vi "Change Database.vi"(8 "error in (no error)":errorcluster, 11 "Node Ptr":u64 format="%.0x") -> (0 "error out":errorcluster)   [LabVIEW 2025, in "Protection and Counter Addon System Explorer.lvlib"]
uses:
  Protection and Counter Addon System Explorer.lvlib
  Types/Base Frame Info.ctl
  <vilib>/NI VeriStand/Custom Device API/Custom Device Item Ref.ctl
  Types/CAN Filter Type.ctl
  <vilib>/NI VeriStand/Custom Device Tools/Custom Device Utility Library/Search Direction.ctl
  <vilib>/NI VeriStand/Custom Device API/Custom Device Channel.ctl
  <vilib>/NI VeriStand/Custom Device API/Custom Device Channel Type.ctl
  Addon Shared/SubVIs/GUID Lookup.vi
  <vilib>/NI/NI VeriStand Advanced SysDef API/_SubVIs/SysDef.Search.GUIDs.vi
  <vilib>/NI VeriStand/Custom Device API/Get Item Property (U32).vi
  <vilib>/NI VeriStand/Custom Device Tools/Custom Device Utility Library/NI VeriStand - Search for Item by GUID.vi
  <vilib>/NI/NI VeriStand Advanced SysDef API/_SubVIs/SysDef.Property.Set.U32.vi
  <vilib>/NI/NI VeriStand Advanced SysDef API/_SubVIs/SysDef.Search.Name.vi
  Addon Shared/Protection and Counter Addon Shared.lvlib
  <vilib>/NI/NI VeriStand Advanced SysDef API/SysDef API/Advanced System Definition.lvlib
  <vilib>/NI VeriStand/Custom Device API/Custom Device API.lvlib
  <resource>/objmgr/xnet.rc
  <vilib>/NI VeriStand/Custom Device Tools/Custom Device Utility Library/Custom Device Utility Library.lvlib
panel:
  in  "Tag":string
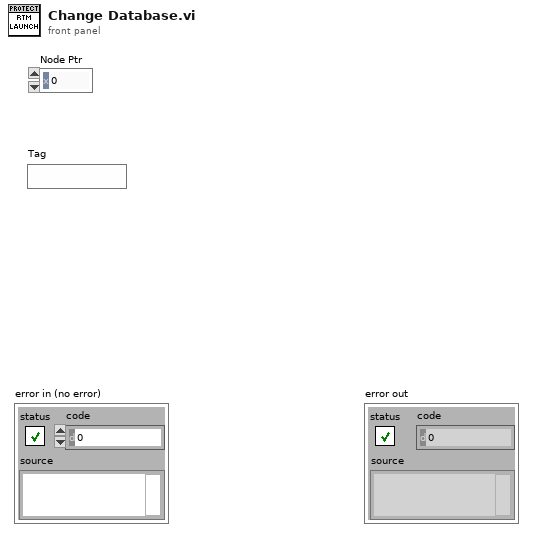
[diagram p1: front panel]
types:
  T1 = typedef "Protection and Counter Addon System Explorer.lvlib/Base Frame Info.ctl" = cluster{"Name":string, "ID":u32, "Signals":string[], "Node Ref":T2, "Type":T3}
  T2 = typedef "Custom Device API.lvlib/Custom Device Item Ref.ctl" = u64
  T3 = typedef "Protection and Counter Addon System Explorer.lvlib/CAN Filter Type.ctl" = enum16{"Cyclic Data", "Event Data", "Cyclic/Event", "All"}
  T4 = typedef "Custom Device API.lvlib/Custom Device Item Info.ctl" = cluster{"Name":string, "Is Channel":bool, "GUID":string, "Is Waveform":bool}
  T5 = typedef "Protection and Counter Addon Shared.lvlib/XNET Settings.ctl" = cluster{"Database":refnum<k21>, "Cluster":refnum<k21>, "Port":string, "Baud rate [Bd]":u64, "Termination":u32, "CAN I/O Mode":u32, "FD Baud rate [Bd]":u64, "Priority":i32, "Use Legacy":bool, "FD ISO Mode":u32, "Default Max Counter Value":dbl, "Default Protect Type":T6}
  T6 = typedef "Protection and Counter Support Shared.lvlib/Protection Type.ctl" = enum16{"Arb ID + Bytes Checksum with Inversion", "Arb ID + Bytes CRC with Inversion", "Reversed Raw Signal Checksum with Inversion", "Concatenated Two's Compliment"}
  T7 = typedef "Protection and Counter Addon System Explorer.lvlib/CAN Update Results.ctl" = cluster{"Frames to Delete":T2[], "Frames to Update":T8[], "New Cluster":refnum<k21>, "Frames to Add":T9[]}
  T8 = typedef "Protection and Counter Addon System Explorer.lvlib/CAN Frame Update Results.ctl" = cluster{"Node Ref":T2, "Name":string, "ID":u32, "New Signals":string[], "Delete Signals":string[], "Type":T3}
  T9 = typedef "Protection and Counter Addon System Explorer.lvlib/Base Frame Info_NoVS.ctl" = cluster{"Name":string, "ID":u32, "Signals":string[], "Type":T3}
  T10 = typedef "Custom Device Utility Library.lvlib/Search Direction.ctl" = enum16{"Down", "Up"}
  T11 = typedef "Custom Device API.lvlib/Custom Device Channel.ctl" = cluster{"Type":T12, "Units":string, "Default Value":dbl, "Faultable":bool, "Scalable":bool}
  T12 = typedef "Custom Device API.lvlib/Custom Device Channel Type.ctl" = enum16{"Input", "Output"}
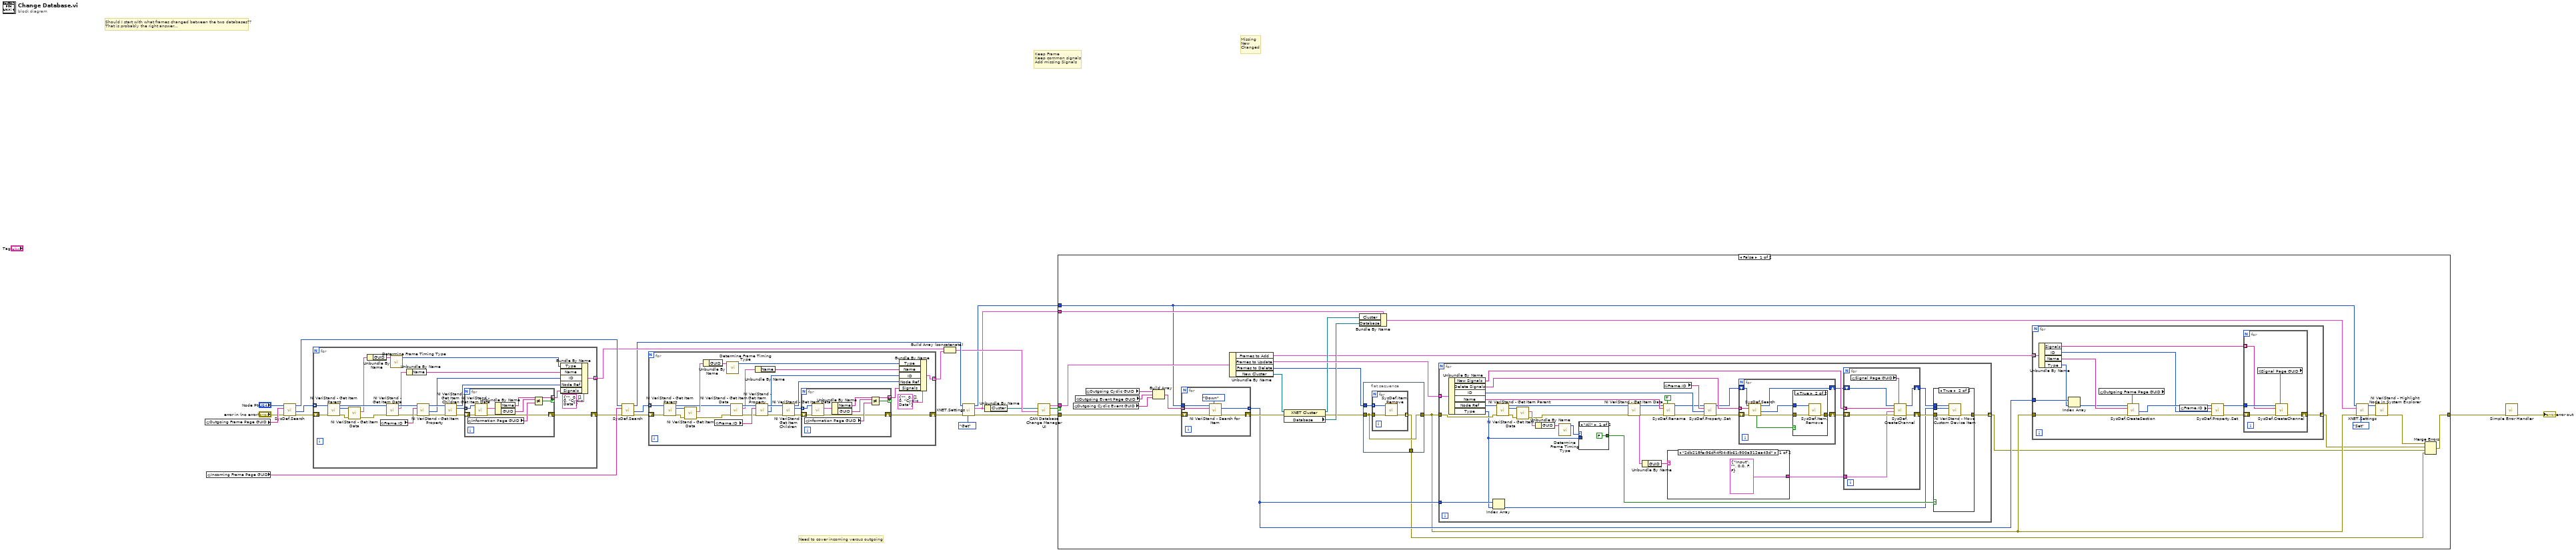
[diagram p0: block diagram]
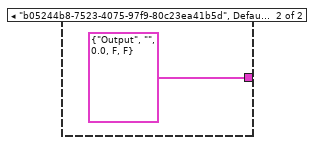
[diagram p4: hidden frame]
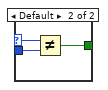
[diagram p5: hidden frame]
diagram:
  # "Missing\nNew\nChanged"
  # "Should I start with what frames changed between the two databases??\nThat is probably the right answer..."
  # "Keep Frame\nKeep common signals\nAdd missing Signals"
  # "Need to cover incoming versus outgoing"
  n1 = global read "GUID Lookup.vi" "Outgoing Frame Page GUID"() -> (w25:string)
  n2 = global read "GUID Lookup.vi" "Incoming Frame Page GUID"() -> (w24:string)
  n3 = call-poly <vilib>:"SysDef.Search.vi"("error in (no error)"="error in (no error)", "GUID"=w25, "nodeID"="Node Ptr") -> ("error out"=w23:errorcluster, "Values Out"=w22:u64[], "nodeID out"=w18:u64)  [unwired: 5 in, 1 out]
  n4 = for {
    tunnel: w22 -> [w33] mode=indexing
    tunnel: [w39] -> w17 mode=indexing
    shift-right: [w38] -> w19
    shift-left: w23 -> [w32]
    n5 = call <vilib>:"NI VeriStand - Get Item Parent.vi"("error in (no error)"=w32, "Item Ref in"=w33) -> ("error out"=w30:errorcluster, "Parent Ref"=w31:T2, "Item Ref out"=w34:T2)  [unwired: 6 in, 1 out]
    n6 = call <vilib>:"NI VeriStand - Get Item Data.vi"("error in (no error)"=w30, "Item Ref in"=w31) -> ("error out"=w29:errorcluster, "Item Info"=w28:T4)  [unwired: 6 in, 2 out]
    n7 = Unbundle By Name(w28) -> ("GUID"=w27:string)
    n8 = global read "GUID Lookup.vi" "Frame.ID"() -> (w47:string)
    n9 = call <vilib>:"NI VeriStand - Get Item Data.vi"("error in (no error)"=w29, "Item Ref in"=w34) -> ("error out"=w44:errorcluster, "Item Info"=w42:T4, "Item Ref out"=w43:T2)  [unwired: 6 in, 1 out]
    n10 = call "Determine Frame Timing Type.vi"("GUID"=w27) -> ("CAN:Frame Type"=w26:T3)  [unwired: 10 in]
    n11 = Unbundle By Name(w42) -> ("Name"=w36:string)
    n12 = call-poly <vilib>:"NI VeriStand - Get Item Property.vi"("error in (no error)"=w44, "Property Name"=w47, "Item Ref in"=w43) -> ("error out"=w48:errorcluster, "Value"=w41:u32, "Item Ref out"=w49:T2)  [unwired: 5 in, 1 out]
    n13 = call <vilib>:"NI VeriStand - Get Item Children.vi"("error in (no error)"=w48, "Item Ref in"=w49) -> ("error out"=w45:errorcluster, "Child Refs"=w46:T2[], "Item Ref out"=w35:T2)  [unwired: 6 in, 1 out]
    n14 = for {
      tunnel: w46 -> [w57] mode=indexing
      shift-right: [w52] -> w38
      shift-left: w45 -> [w56]
      tunnel: [w50] -> w40 mode=indexing if=w51
      n15 = global read "GUID Lookup.vi" "Information Page GUID"() -> (w54:string)
      n16 = call <vilib>:"NI VeriStand - Get Item Data.vi"("error in (no error)"=w56, "Item Ref in"=w57) -> ("error out"=w52:errorcluster, "Item Info"=w55:T4)  [unwired: 6 in, 2 out]
      n17 = Unbundle By Name(w55) -> ("Name"=w50:string, "GUID"=w53:string)
      n18 = Not Equal?(x=w53, y=w54) -> (x != y?=w51:bool)
    }
    n19 = Bundle By Name(cluster=T1 {"Name"="", "ID"=0, "Signals"=[], "Node Ref"=0, "Type"=enum."Cyclic Data"}, "Type"=w26, "Name"=w36, "ID"=w41, "Node Ref"=w35, "Signals"=w40) -> (w39:T1)
  }
  n20 = call-poly <vilib>:"SysDef.Search.vi"("error in (no error)"=w19, "GUID"=w24, "nodeID"=w18) -> ("error out"=w20:errorcluster, "Values Out"=w21:u64[], "nodeID out"=w8:u64)  [unwired: 5 in, 1 out]
  n21 = for {
    tunnel: w21 -> [w61] mode=indexing
    shift-right: [w70] -> w9
    shift-left: w20 -> [w62]
    tunnel: [w69] -> w16 mode=indexing
    n22 = call <vilib>:"NI VeriStand - Get Item Parent.vi"("error in (no error)"=w62, "Item Ref in"=w61) -> ("error out"=w65:errorcluster, "Parent Ref"=w66:T2, "Item Ref out"=w59:T2)  [unwired: 6 in, 1 out]
    n23 = call <vilib>:"NI VeriStand - Get Item Data.vi"("error in (no error)"=w65, "Item Ref in"=w66) -> ("error out"=w60:errorcluster, "Item Info"=w64:T4)  [unwired: 6 in, 2 out]
    n24 = Unbundle By Name(w64) -> ("GUID"=w63:string)
    n25 = global read "GUID Lookup.vi" "Frame.ID"() -> (w79:string)
    n26 = call "Determine Frame Timing Type.vi"("GUID"=w63) -> ("CAN:Frame Type"=w58:T3)  [unwired: 10 in]
    n27 = call <vilib>:"NI VeriStand - Get Item Data.vi"("error in (no error)"=w60, "Item Ref in"=w59) -> ("error out"=w78:errorcluster, "Item Info"=w72:T4, "Item Ref out"=w76:T2)  [unwired: 6 in, 1 out]
    n28 = Unbundle By Name(w72) -> ("Name"=w71:string)
    n29 = call-poly <vilib>:"NI VeriStand - Get Item Property.vi"("error in (no error)"=w78, "Property Name"=w79, "Item Ref in"=w76) -> ("error out"=w77:errorcluster, "Value"=w73:u32, "Item Ref out"=w75:T2)  [unwired: 5 in, 1 out]
    n30 = call <vilib>:"NI VeriStand - Get Item Children.vi"("error in (no error)"=w77, "Item Ref in"=w75) -> ("error out"=w80:errorcluster, "Child Refs"=w81:T2[], "Item Ref out"=w67:T2)  [unwired: 6 in, 1 out]
    n31 = for {
      tunnel: w81 -> [w89] mode=indexing
      shift-right: [w84] -> w70
      shift-left: w80 -> [w88]
      tunnel: [w82] -> w74 mode=indexing if=w83
      n32 = global read "GUID Lookup.vi" "Information Page GUID"() -> (w86:string)
      n33 = call <vilib>:"NI VeriStand - Get Item Data.vi"("error in (no error)"=w88, "Item Ref in"=w89) -> ("error out"=w84:errorcluster, "Item Info"=w87:T4)  [unwired: 6 in, 2 out]
      n34 = Unbundle By Name(w87) -> ("Name"=w82:string, "GUID"=w85:string)
      n35 = Not Equal?(x=w85, y=w86) -> (x != y?=w83:bool)
    }
    n36 = Bundle By Name(cluster=T1 {"Name"="", "ID"=0, "Signals"=[], "Node Ref"=0, "Type"=enum."Cyclic Data"}, "Type"=w58, "Name"=w71, "ID"=w73, "Node Ref"=w67, "Signals"=w74) -> (w69:T1)
  }
  n37 = Build Array (concatenate)(w17, w16) -> (w6:T1[])
  n38 = call "XNET.Settings.vi"("Action"=enum8{"Get", "Set"}."Get", "error in (no error)"=w9, "Parent Ref in"=w8) -> ("error out"=w5:errorcluster, "XNET Settings"=w3:T5, "Item Ref out"=w2:T2)  [unwired: 6 in]
  n39 = Unbundle By Name(w3) -> ("Cluster"=w4:refnum<k21>)
  n40 = call "CAN Database Change Manager UI.vi"("error in (no error)"=w5, "VS Existing Frames"=w6, "Old Cluster"=w4) -> ("error out"=w13:errorcluster, "Cancel Out"=w12:bool, "CAN Update"=w11:T7)  [unwired: 6 in]
  n41 = case shown="False" w12 {
    tunnel: w13 -> [w101 w213]
    tunnel: w11 -> [w116 _]
    tunnel: [w90 w213] -> w10
    tunnel: w3 -> [w113 _]
    tunnel: w2 -> [w104 _]
    frame False {
      n42 = global read "GUID Lookup.vi" "Outgoing Cyclic Event GUID"() -> (w105:string)
      n43 = global read "GUID Lookup.vi" "Outgoing Event Page GUID"() -> (w106:string)
      n44 = global read "GUID Lookup.vi" "Outgoing Cyclic GUID"() -> (w107:string)
      n45 = Build Array(w107, w106, w105) -> (w103:string[])
      n46 = for {
        tunnel: w104 -> [w127]
        tunnel: w103 -> [w126] mode=indexing
        shift-right: [w124] -> w102
        shift-left: w101 -> [w125]
        tunnel: [w123] -> w97 mode=indexing
        n47 = call-poly <vilib>:"NI VeriStand - Search for Item.vi"("Direction (Down)"=Search_Direction."Down", "error in"=w125, "Item GUID"=w126, "Section Ref in"=w127) -> ("error out"=w124:errorcluster, "Item Ref"=w123:T2)  [unwired: 4 in, 2 out]
      }
      n48 = Unbundle By Name(w116) -> ("Frames to Add"=w98:T9[], "Frames to Update"=w115:T8[], "Frames to Delete"=w99:T2[], "New Cluster"=w100:refnum<k21>)
      n49 = property class="XNET Cluster"(reference=w100, error in=w102) -> (reference out=w112:refnum<k21>, error out=w96:errorcluster, "Database"=w111:refnum<k21>)
      n50 = Bundle By Name(cluster=w113, "Cluster"=w112, "Database"=w111) -> (w110:T5)
      n51 = flat-sequence {
        tunnel: w99 -> [w119]
        tunnel: w96 -> [w118]
        tunnel: [w118] -> w95
        tunnel: [w117] -> w92
        frame #0 {
          n52 = for {
            tunnel: w119 -> [w120] mode=indexing
            tunnel: w118 -> [w122]
            tunnel: [w121] -> w117 mode=indexing
            n53 = call <vilib>:"SysDef.Item.Remove.vi"("error in (no error)"=w122, "nodeID"=w120) -> ("error out"=w121:errorcluster)  [unwired: 8 in, 1 out]
          }
        }
      }
      n54 = for {
        tunnel: w115 -> [w162] mode=indexing
        tunnel: w97 -> [w147]
        tunnel: w95 -> [w150]
        tunnel: [w132] -> w93 mode=indexing
        n55 = Unbundle By Name(w162) -> ("New Signals"=w157:string[], "Delete Signals"=w158:string[], "ID"=w160:u32, "Name"=w161:string, "Node Ref"=w152:T2, "Type"=w146:T3)
        n56 = Index Array(array=w147, index=w146) -> (element=w130:T2)
        n57 = call <vilib>:"NI VeriStand - Get Item Parent.vi"("error in (no error)"=w150, "Item Ref in"=w152) -> ("error out"=w155:errorcluster, "Parent Ref"=w156:T2, "Item Ref out"=w151:T2)  [unwired: 6 in, 1 out]
        n58 = call <vilib>:"NI VeriStand - Get Item Data.vi"("error in (no error)"=w155, "Item Ref in"=w156) -> ("error out"=w149:errorcluster, "Item Info"=w154:T4)  [unwired: 6 in, 2 out]
        n59 = Unbundle By Name(w154) -> ("GUID"=w153:string)
        n60 = call "Determine Frame Timing Type.vi"("GUID"=w153) -> ("CAN:Frame Type"=w148:T3)  [unwired: 10 in]
        n61 = case shown="\"All\"" w148 {
          selector: w148 -> [_ w190]
          tunnel: w146 -> [_ w192]
          tunnel: [FALSE w191] -> w131
          frame "All" {
          }
          frame Default {
            n62 = Not Equal?(x=w190, y=w192) -> (x != y?=w191:bool)
          }
        }
        n63 = call <vilib>:"NI VeriStand - Get Item Data.vi"("error in (no error)"=w149, "Item Ref in"=w151) -> ("error out"=w139:errorcluster, "Item Info"=w138:T4, "Item Ref out"=w140:T2)  [unwired: 6 in, 1 out]
        n64 = Unbundle By Name(w138) -> ("GUID"=w137:string)
        n65 = call <vilib>:"SysDef.Rename.vi"("Force Rename (F)"=TRUE, "error in (no error)"=w139, "Name"=w161, "nodeID"=w140) -> ("error out"=w144:errorcluster, "nodeID out"=w145:u64)  [unwired: 5 in, 1 out]
        n66 = global read "GUID Lookup.vi" "Frame.ID"() -> (w159:string)
        n67 = case shown="\"2db218fe-96df-4f04-8b61-900a312ea43d\"" w137 {
          tunnel: [T11 {"Type"=enum."Input", "Units"="", "Default Value"=0.0, "Faultable"=FALSE, "Scalable"=FALSE} ("Channel") T11 {"Type"=enum."Output", "Units"="", "Default Value"=0.0, "Faultable"=FALSE, "Scalable"=FALSE} ("Channel")] -> w136
          frame "2db218fe-96df-4f04-8b61-900a312ea43d" {
          }
          frame "b05244b8-7523-4075-97f9-80c23ea41b5d", Default {
          }
        }
        n68 = call-poly <vilib>:"SysDef.Property.Set.vi"("error in (no error)"=w144, "Value"=w160, "Property Name"=w159, "nodeID"=w145) -> ("error out"=w135:errorcluster, "nodeID out"=w143:u64)  [unwired: 6 in]
        n69 = for {
          tunnel: w158 -> [w175] mode=indexing
          shift-right: [w178] -> w142
          shift-left: w143 -> [w182]
          shift-right: [w177] -> w141
          shift-left: w135 -> [w176]
          n70 = call-poly <vilib>:"SysDef.Search.vi"("error in (no error)"=w176, "Name"=w175, "nodeID"=w182) -> ("error out"=w179:errorcluster, "Value out"=w180:u64, "nodeID out"=w178:u64, "Found?"=w181:bool)  [unwired: 5 in]
          n71 = case shown="True" w181 {
            tunnel: w180 -> [_ w186]
            tunnel: w179 -> [w183 w185]
            tunnel: [w183 w184] -> w177
            frame False {
            }
            frame True {
              n72 = call <vilib>:"SysDef.Item.Remove.vi"("error in (no error)"=w185, "nodeID"=w186) -> ("error out"=w184:errorcluster)  [unwired: 8 in, 1 out]
            }
          }
        }
        n73 = for {
          tunnel: w136 -> [w171]
          shift-right: [w170] -> w133
          shift-left: w141 -> [w173]
          tunnel: w157 -> [w169] mode=indexing
          shift-right: [w168] -> w129
          shift-left: w142 -> [w174]
          n74 = global read "GUID Lookup.vi" "Signal Page GUID"() -> (w172:string)
          n75 = call <vilib>:"SysDef.CreateChannel.vi"("GUID"=w172, "error in (no error)"=w173, "Channel"=w171, "Name"=w169, "nodeID"=w174) -> ("error out"=w170:errorcluster, "nodeID out"=w168:u64)  [unwired: 3 in, 2 out]
        }
        n76 = case shown="True" w131 {
          tunnel: w133 -> [w163 w167]
          tunnel: w129 -> [_ w165]
          tunnel: [w163 w166] -> w132
          tunnel: w130 -> [_ w164]
          frame False {
          }
          frame True {
            n77 = call <vilib>:"NI VeriStand - Move Custom Device Item.vi"("error in (no error)"=w167, "New Parent Ref in"=w164, "Item Ref in"=w165) -> ("error out"=w166:errorcluster)  [unwired: 6 in, 2 out]
          }
        }
      }
      n78 = for {
        tunnel: w98 -> [w207] mode=indexing
        tunnel: w97 -> [w206]
        tunnel: w95 -> [w194]
        tunnel: [w193] -> w94 mode=indexing
        n79 = Unbundle By Name(w207) -> ("Signals"=w198:string[], "ID"=w203:u32, "Name"=w201:string, "Type"=w205:T3)
        n80 = Index Array(array=w206, index=w205) -> (element=w195:T2)
        n81 = global read "GUID Lookup.vi" "Outgoing Frame Page GUID"() -> (w196:string)
        n82 = call <vilib>:"SysDef.CreateSection.vi"("GUID"=w196, "error in (no error)"=w194, "Name"=w201, "nodeID"=w195) -> ("error out"=w202:errorcluster, "New NodeID"=w204:u64)  [unwired: 4 in, 2 out]
        n83 = global read "GUID Lookup.vi" "Frame.ID"() -> (w197:string)
        n84 = call-poly <vilib>:"SysDef.Property.Set.vi"("error in (no error)"=w202, "Value"=w203, "Property Name"=w197, "nodeID"=w204) -> ("error out"=w199:errorcluster, "nodeID out"=w200:u64)  [unwired: 6 in]
        n85 = for {
          tunnel: w200 -> [w212]
          tunnel: w198 -> [w210] mode=indexing
          shift-right: [w209] -> w193
          shift-left: w199 -> [w211]
          n86 = global read "GUID Lookup.vi" "Signal Page GUID"() -> (w208:string)
          n87 = call <vilib>:"SysDef.CreateChannel.vi"("GUID"=w208, "error in (no error)"=w211, "Name"=w210, "nodeID"=w212) -> ("error out"=w209:errorcluster)  [unwired: 4 in, 3 out]
        }
      }
      n88 = call "XNET.Settings.vi"("Action"=enum8{"Get", "Set"}."Set", "error in (no error)"=w95, "XNET Settings"=w110, "Parent Ref in"=w104) -> ("error out"=w109:errorcluster, "Item Ref out"=w108:T2)  [unwired: 5 in, 1 out]
      n89 = call <vilib>:"NI VeriStand - Highlight Node in System Explorer.vi"("error in (no error)"=w109, "Item Ref in"=w108) -> ("error out"=w91:errorcluster)  [unwired: 8 in, 1 out]
      n90 = Merge Errors(w91, w94, w93, w92) -> (w90:errorcluster)
    }
    frame True {
    }
  }
  n91 = call <vilib>:"Simple Error Handler.vi"("error in (no error)"=w10) -> ("error out"=→"error out":errorcluster)  [unwired: 4 in, 4 out]
